vi "Gen_ctrl.vi"(8 "error in (no error)":errorcluster, 9 "Controller On?":bool, 10 "Kp":dbl=1.0, 11 "Error In":dbl) -> (0 "error out":errorcluster, 3 "Ctrl Effort Out":dbl)   [LabVIEW 2018, in "Controller.lvlib"]
doc: "Generic Discrete-time controller"
uses:
  Controller.lvlib
  <vilib>/Simulation/Shared/_Datatypes/SIM SISO Transfer Function.ctl
  <vilib>/Simulation/DiscreteLinear/Implementation/NILVSim Discrete Transfer Function Direct.llb/SIM Discrete Transfer Function Diagram (SISO).vi
  <vilib>/Simulation/ContinuousLinear/Implementation/Shared/SIM Transfer Function Support.llb/SIM TransferFunction Normalize to Buffer.vi
  <vilib>/Simulation/DiscreteLinear/Implementation/Shared/SIM Init Discrete States.vi
  <vilib>/Simulation/DiscreteLinear/Implementation/NILVSim Discrete Transfer Function Direct.llb/SIM Transfer Function Direct core (SISO).vi
  <vilib>/Simulation/ContinuousLinear/Implementation/Shared/SIM Transfer Function Support.llb/SIM TransferFunction Normalize.vi
  <vilib>/Simulation/Implementation/Shared/SIM Polynomials.llb/SIM Remove Zero Coefficients (DBL).vi
  <vilib>/Simulation/Implementation/Shared/SIM Polynomials.llb/SIM Divide Polynomials (DBL).vi
  <vilib>/Simulation/Implementation/Shared/SIM BuildSimErr.vi
  <vilib>/Simulation/Implementation/XNodeFramework/SimXNode/SimX.xnode
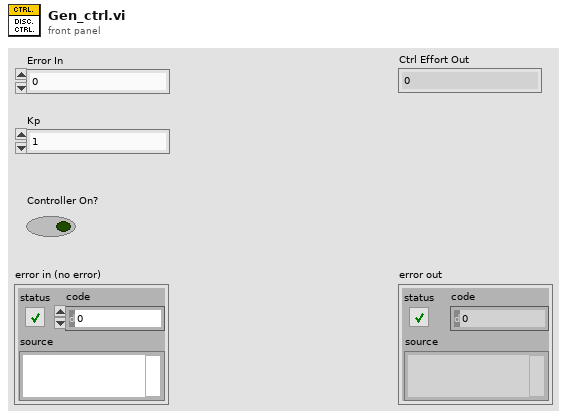
[diagram p1: front panel]
types:
  T1 = typedef "SIM SISO Transfer Function.ctl" = cluster{"Numerator":dbl[], "Denominator":dbl[]}
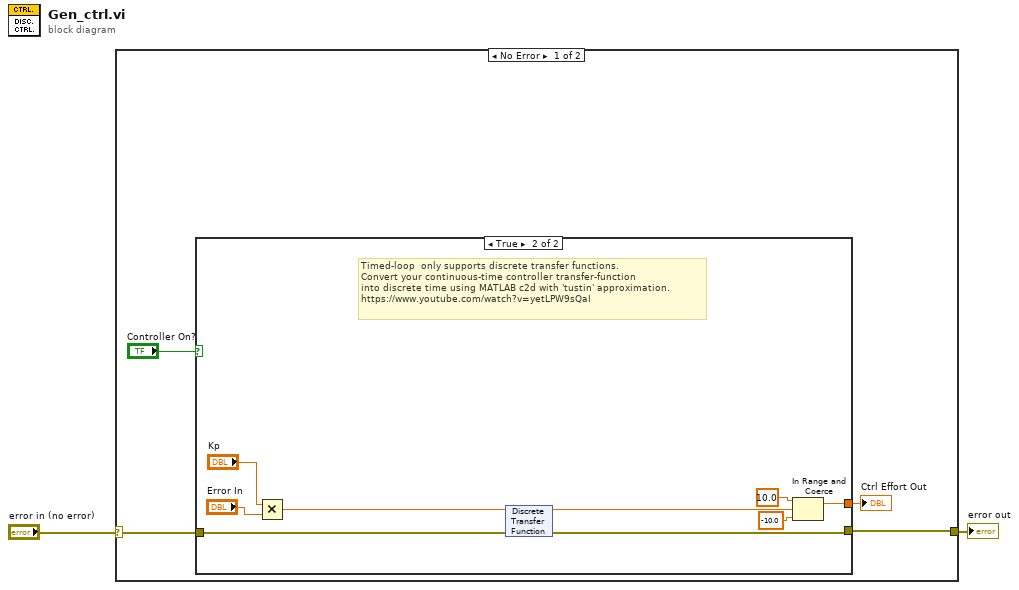
[diagram p0: block diagram]
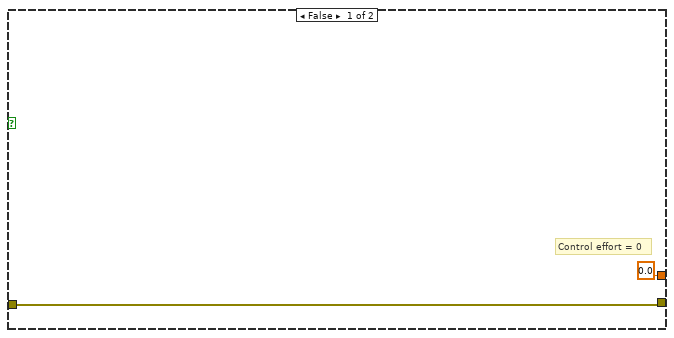
[diagram p2: hidden frame]
diagram:
  n1 = case shown="No Error" "error in (no error)" {
    selector: "error in (no error)" -> [w6 w24]
    tunnel: [w5 w24] -> w1
    frame No Error {
      n2 = case shown="True" "Controller On?" {
        tunnel: w6 -> [w7 w10]
        tunnel: [w7 w9] -> w5
        tunnel: [0.0 ("upper limit") w15] -> w3
        frame False {
          # "Control effort = 0"
        }
        frame True {
          # "Timed-loop  only supports discrete transfer functions.\nConvert your continuous-time controller transfer-function \ninto discrete time using MATLAB c2d with 'tustin' approximation.\nhttps://www.youtube.com/watch?v=yetLPW9sQaI"
          n3 = Multiply(x="Kp", y="Error In") -> (x*y=w12:dbl)
          n4 = xnode "Discrete Transfer Function"("input u(k)"=w12, "error in (no error)"=w10) -> ("output y(k)"=w11:dbl, "error out"=w9:errorcluster)  [unwired: 1 in]
          n5 = In Range and Coerce(upper limit=10.0, x=w11, lower limit=-10.0) -> (coerced(x)=w15:dbl)  [unwired: 1 out]
        }
      }
      "Ctrl Effort Out" <- w3
    }
    frame Error {
    }
  }
  "error out" <- w1
